vi "Read Filter Type.vi"(8 "error in (no error)":errorcluster, 11 "Filter in":refnum<class "Filter.lvclass">) -> (0 "error out":errorcluster, 2 "Command Type":T1, 3 "Filter out":refnum<class "Filter.lvclass">)   [LabVIEW 2020, in "BCI-1553 API.lvlib" / "Filter.lvclass"]
uses:
  Filter.lvclass
  Frames & Messages/TypeDefs/Command Type.ctl
  Filter.lvclass/Filter.ctl
  BCI-1553 API.lvlib
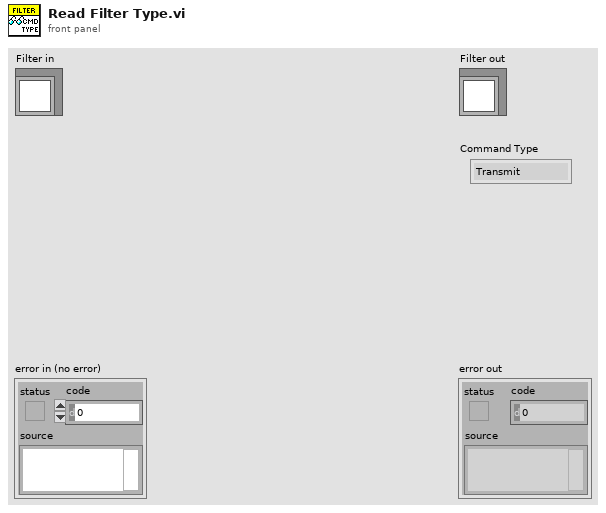
[diagram p1: front panel]
types:
  T1 = typedef "BCI-1553 API.lvlib/Command Type.ctl" = enum16{"Transmit", "Receive"}
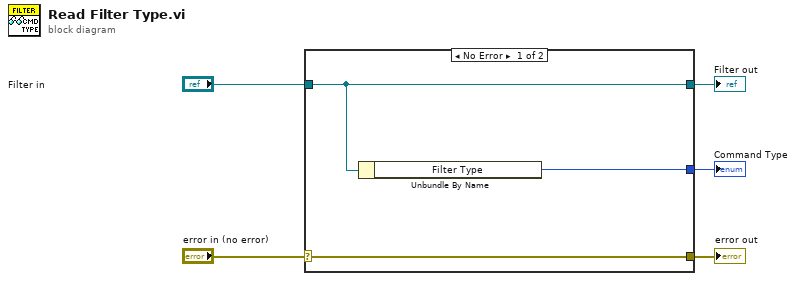
[diagram p0: block diagram]
diagram:
  n1 = case shown="No Error" "error in (no error)" {
    selector: "error in (no error)" -> [w8 w9]
    tunnel: [w8 w9] -> w4
    tunnel: [w7 w10] -> w2
    tunnel: "Filter in" -> [w7 w10]
    tunnel: [w6 _] -> w1
    frame No Error {
      n2 = Unbundle By Name(w7) -> ("Filter Type"=w6:T1)
    }
    frame Error {
    }
  }
  "error out" <- w4
  "Filter out" <- w2
  "Command Type" <- w1
